vi "Graph Handler.vi"(0 "WF Ref Array":refnum<vi>[](array[refnum]), 2 "State":string, 7 "Data":dbl[](array[numeric]), 9 "ChSize":i32=1, 11 "NumCh":i32=1) -> ()   [LabVIEW 2013]
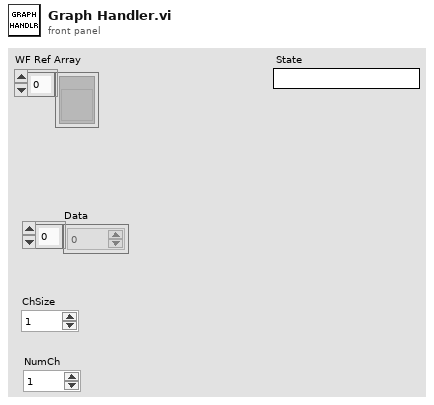
[diagram p1: front panel]
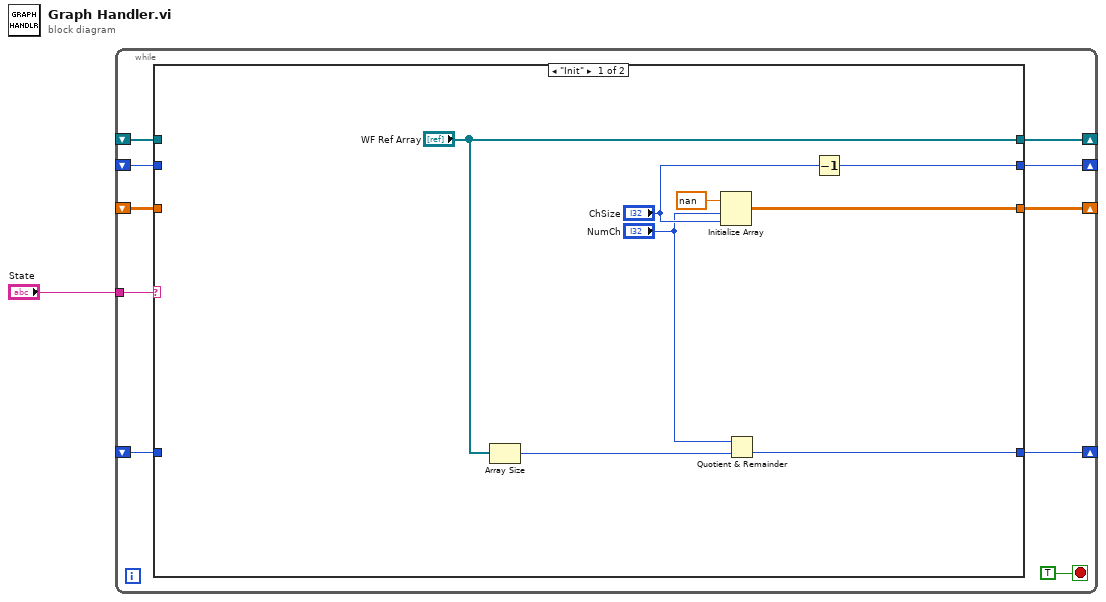
[diagram p0: block diagram]
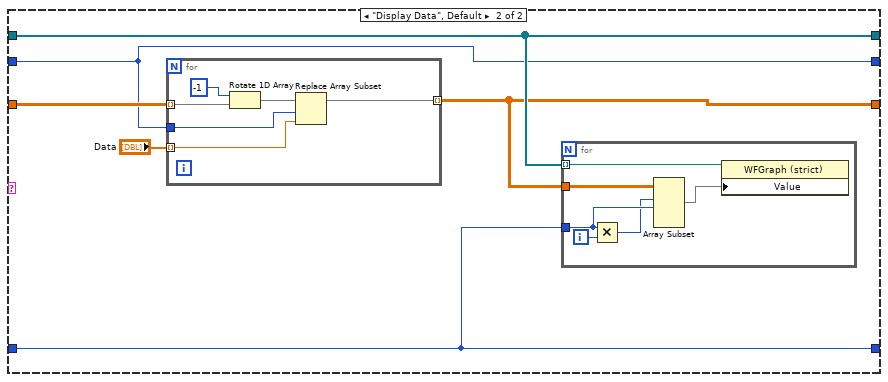
[diagram p2: hidden frame]
diagram:
  n1 = while {
    tunnel: "State" -> [w10]
    shift-right: [w8] -> _
    shift-left: _ -> [w7]
    shift-right: [w9] -> _
    shift-left: _ -> [w6]
    shift-right: [w5] -> _
    shift-left: _ -> [w4]
    shift-right: [w3] -> _
    shift-left: _ -> [w2]
    stop <- TRUE stop-if-true
    n2 = case shown="\"Init\"" w10 {
      tunnel: [w19 w22] -> w9
      tunnel: ["WF Ref Array" w23] -> w8
      tunnel: w7 -> [_ w23]
      tunnel: w6 -> [_ w25]
      tunnel: [w18 w20] -> w5
      tunnel: w4 -> [_ w20]
      tunnel: [w14 w21] -> w3
      tunnel: w2 -> [_ w21]
      frame "Init" {
        n3 = Array Size(array="WF Ref Array") -> (size(s)=w13:i32)
        n4 = Initialize Array(nan, "NumCh", "ChSize") -> (w19:dbl[][])
        n5 = Quotient & Remainder(x="NumCh", y=w13) -> (floor(x/y)=w14:i32)  [unwired: 1 out]
        n6 = Decrement(x="ChSize") -> (x-1=w18:i32)
      }
      frame "Display Data", Default {
        n7 = for {
          tunnel: w25 -> [w36] mode=indexing
          tunnel: w20 -> [w34]
          tunnel: [w32] -> w22 mode=indexing
          tunnel: "Data" -> [w33] mode=indexing
          n8 = Rotate 1D Array(1:w36, 2:-1 ("n")) -> (0:w35:dbl[])
          n9 = Replace Array Subset(array=w35, new element=w33, index=w34) -> (w32:dbl[])
        }
        n10 = for {
          tunnel: w23 -> [w31] mode=indexing
          tunnel: w22 -> [w30]
          tunnel: w21 -> [w27]
          i -> [w29]
          n11 = Multiply(x=w27, y=w29) -> (x*y=w26:i32)
          n12 = Array Subset(array=w30, index (row)=w26, length (row)=w27) -> (w28:dbl[][])  [unwired: 2 in]
          n13 = property class="WFGraph (strict)"(reference=w31, "Value"=w28) -> ()  [unwired: 1 in, 2 out]
        }
      }
    }
  }
